vi "SEARCH_FOR_GOAL.vi"(10 "argv":string[](array[string]), 11 "args":u8) -> ()   [LabVIEW 2015]
uses:
  Team Code/Robot Global Data.vi
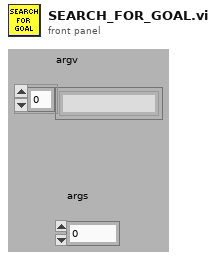
[diagram p1: front panel]
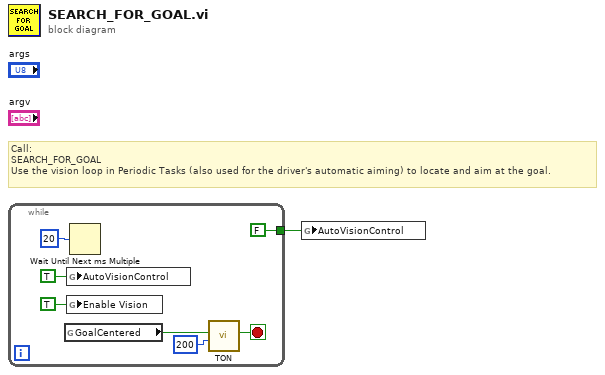
[diagram p0: block diagram]
diagram:
  # "Call:\nSEARCH_FOR_GOAL\nUse the vision loop in Periodic Tasks (also used for the driver's automatic aiming) to locate and aim at the goal."
  n1 = while {
    tunnel: [FALSE] -> w1
    stop <- w3 stop-if-true
    n2 = global read "Robot Global Data.vi" "GoalCentered"() -> (w4:bool)
    n3 = global write "Robot Global Data.vi" "AutoVisionControl"(TRUE ("Enable Vision")) -> ()
    n4 = global write "Robot Global Data.vi" "Enable Vision"(TRUE ("Enable Vision")) -> ()
    n5 = Wait Until Next ms Multiple(millisecond multiple=u32 20) -> ()  [unwired: 1 out]
    n6 = call "TON.vi"("Delay (ms)"=u32 200, "Input"=w4) -> ("Output"=w3:bool)  [unwired: 9 in]
  }
  n7 = global write "Robot Global Data.vi" "AutoVisionControl"(w1) -> ()
